vi "Configure AI.vi"(8 "error in":errorcluster, 10 "AI Channel":tag, 11 "DAQ HVPS in":refnum<class "DAQ HVPS.lvclass">) -> (0 "error out":errorcluster, 3 "DAQ HVPS out":refnum<class "DAQ HVPS.lvclass">)   [LabVIEW 2013, in "DAQ HVPS.lvclass"]
doc: "Define a scale called <b>HVPS Scale</b> that is 0 to 5kV and uses a multiplier of 500 to convert acquired voltage to the actual HVPS voltage. We will acquire a finite number of samples at a rate 1 kHz (over 100 ms). Configuring the channel liek this instead of as a continuous acquisition device prevents us from having to properly handle opening and closing the connection to the channel. The channel is set to autostart."
uses:
  DAQ HVPS.lvclass
  DAQ HVPS.lvclass/DAQ HVPS.ctl
  <vilib>/DAQmx/create/scale.llb/DAQmx Create Scale (Linear).vi
  <vilib>/DAQmx/create/channels.llb/DAQmx Create Channel (AI-Voltage-Basic).vi
  <vilib>/DAQmx/configure/timing.llb/DAQmx Timing (Sample Clock).vi
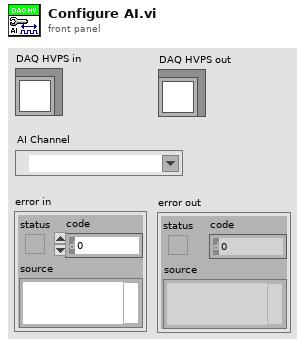
[diagram p1: front panel]
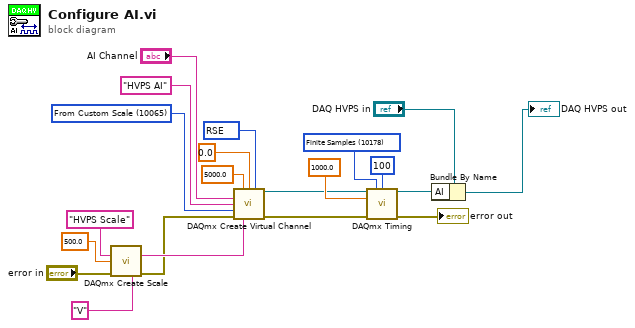
[diagram p0: block diagram]
diagram:
  w4 = 10083 items=["default"=-1, "RSE"=10083, "NRSE"=10078, "Differential"=10106, "Pseudodifferential"=12529] ("input terminal configuration")
  w19 = 10178 items=["Finite Samples"=10178, "Continuous Samples"=10123, "Hardware Timed Single Point"=12522] ("sample mode")
  w16 = 10065 items=["Volts"=10348, "From Custom Scale"=10065] ("units")
  n1 = call-poly <vilib>:"DAQmx Create Scale.vi"("name"="HVPS Scale", "slope"=500.0, "error in"="error in", "scaled units"="V") -> ("scale out"=w8:tag, "error out"=w7:errorcluster)  [unwired: 10 in]
  n2 = call-poly <vilib>:"DAQmx Create Virtual Channel.vi"("maximum value"=5000.0, "minimum value"=0.0, "input terminal configuration"=w4, "physical channels"="AI Channel", "name to assign"="HVPS AI", "units"=w16, "error in"=w7, "custom scale name"=w8) -> ("task out"=w17:refnum<k21>, "error out"=w18:errorcluster)  [unwired: 6 in]
  n3 = call-poly <vilib>:"DAQmx Timing.vi"("task/channels in"=w17, "sample mode"=w19, "samples per channel"=100, "rate"=1000.0, "error in"=w18) -> ("task out"=w2:refnum<k21>, "error out"=→"error out":errorcluster)  [unwired: 9 in]
  n4 = Bundle By Name(cluster="DAQ HVPS in", "AI"=w2) -> (→"DAQ HVPS out":refnum<class "DAQ HVPS.lvclass">)
